vi "action.vi"(0 "NInstrSim_ConfigureWaveformFormat":refnum<class "NInstrSim_ConfigureWaveformFormat.lvclass">, 2 "HGF_Visitable":refnum<class "HGF_Visitable.lvclass">, 5 "error in (no error)":errorcluster) -> (14 "dup NInstrSim_ConfigureWaveformFormat":refnum<class "NInstrSim_ConfigureWaveformFormat.lvclass">, 16 "dup HGF_Visitable":refnum<class "HGF_Visitable.lvclass">, 19 "error out":errorcluster)   [LabVIEW 2009, in "HB_Device_Examples.lvlib" / "NInstrSim_ConfigureWaveformFormat.lvclass"]
doc: "This is a dynamic dispatch VI that is called from Visitor.visit(). It will call member VIs of Visitable to perform the requested action which means: calling public methods of Visitable child class.\n\n<B>Hint:</B> This method is abstract and need to be implemented by child classes."
uses:
  NInstrSim_ConfigureWaveformFormat.lvclass
  lib.lib/HGF_LVC/HGF_BaseClasses/HGF_Visitable/HGF_Visitable.lvclass
  NInstrSim.lvclass
  NInstrSim_ConfigureWaveformFormat.lvclass/NInstrSim_ConfigureWaveformFormat.ctl
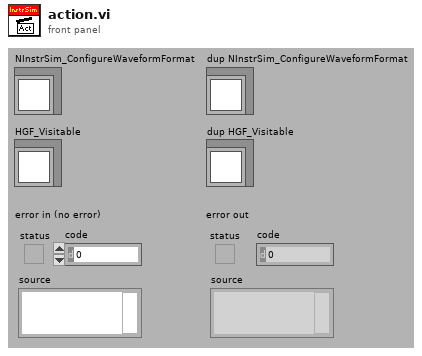
[diagram p1: front panel]
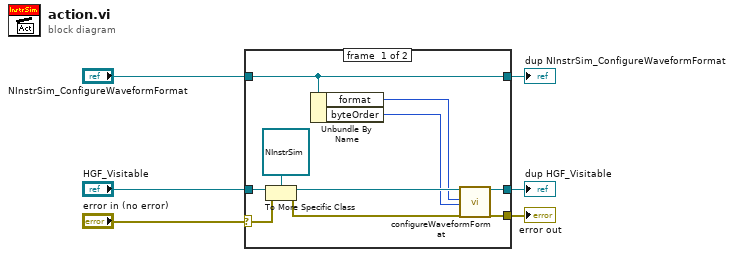
[diagram p0: block diagram]
diagram:
  n1 = case shown="No Error" "error in (no error)" {
    selector: "error in (no error)" -> [w14 w17]
    tunnel: "NInstrSim_ConfigureWaveformFormat" -> [w13 w19]
    tunnel: "HGF_Visitable" -> [w16 w18]
    tunnel: [w11 w18] -> w4
    tunnel: [w9 w17] -> w3
    tunnel: [w13 w19] -> w1
    frame #0 {
      n2 = To More Specific Class(target class=refnum<class "NInstrSim.lvclass"> refnum ("HB_HGF_Test.lvlib:NInstrSim.lvclass"), reference=w16, error in=w14) -> (specific class reference=w12:refnum<class "NInstrSim.lvclass">, error out=w10:errorcluster)
      n3 = Unbundle By Name(w13) -> ("format"=w8:u16, "byteOrder"=w7:u16)
      n4 = call "configureWaveformFormat.vi"("NInstrSim"=w12, "Waveform Format (0:ASCII)"=w8, "Byte Order (0:Low Byte First)"=w7, "error in (no error)"=w10) -> ("dup NInstrSim"=w11:refnum<class "NInstrSim.lvclass">, "error out"=w9:errorcluster)  [unwired: 14 out]
    }
    frame #1 {
    }
  }
  "error out" <- w3
  "dup NInstrSim_ConfigureWaveformFormat" <- w1
  "dup HGF_Visitable" <- w4
